vi "Read Detector Status.vi"(8 "Error In":errorcluster, 11 "KIT-QVA in":refnum<class "KIT-QVA.lvclass">) -> (0 "Error Out":errorcluster, 3 "KIT-QVA out":refnum<class "KIT-QVA.lvclass">)   [LabVIEW 2014, in "KIT-QVA.lvlib" / "KIT-QVA.lvclass"]
doc: "Read detector status and publish."
uses:
  KIT-QVA.lvclass
  KIT-QVA.lvclass/KIT-QVA.ctl
  instr.lib/KIT-QV/KIT QV.lvlib
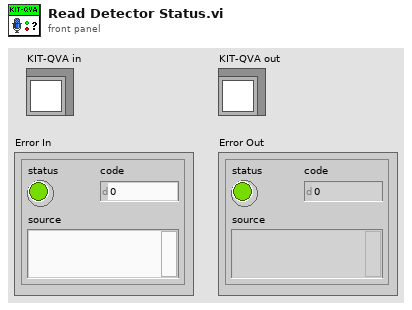
[diagram p1: front panel]
types:
  T1 = cluster{"System Test":bool, "Test Mode":bool, "Fault":bool, "Quench":bool, "U/T Fault":bool, "Bus Error":bool, "System Fault":bool, "Reserved":bool}
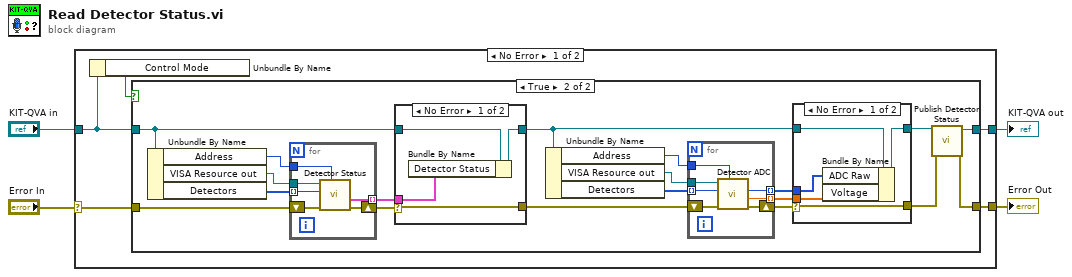
[diagram p0: block diagram]
diagram:
  n1 = case shown="No Error" "Error In" {
    selector: "Error In" -> [w7 w58]
    tunnel: [w8 w58] -> w3
    tunnel: [w9 w57] -> w1
    tunnel: "KIT-QVA in" -> [w6 w57]
    frame No Error {
      n2 = Unbundle By Name(w6) -> ("Control Mode"=w5:bool)
      n3 = case shown="True" w5 {
        tunnel: [w11 w30] -> w9
        tunnel: [w10 w29] -> w8
        tunnel: w7 -> [w10 w28]
        tunnel: w6 -> [w11 w12]
        frame False {
        }
        frame True {
          n4 = Unbundle By Name(w12) -> ("Address"=w25:u16, "VISA Resource out"=w26:refnum<visa-resource-name>, "Detectors"=w23:u8[])
          n5 = for {
            tunnel: w26 -> [w48]
            tunnel: w25 -> [w47]
            tunnel: [w46] -> w24 mode=indexing
            shift-right: [w49] -> w27
            shift-left: w28 -> [w50]
            tunnel: w23 -> [w45] mode=indexing
            n6 = call "Detector Status.vi"("Address"=w47, "Error In"=w50, "Detector"=w45, "VISA Resource in"=w48) -> ("Error Out"=w49:errorcluster, "Detector Cluster"=w46:T1)  [unwired: 4 in, 2 out]
          }
          n7 = case shown="No Error" w27 {
            selector: w27 -> [w51 w55]
            tunnel: w24 -> [w54 _]
            tunnel: w12 -> [w53 w56]
            tunnel: [w52 w56] -> w16
            tunnel: [w51 w55] -> w17
            frame No Error {
              n8 = Bundle By Name(cluster=w53, "Detector Status"=w54) -> (w52:refnum<class "KIT-QVA.lvclass">)
            }
            frame Error {
            }
          }
          n9 = Unbundle By Name(w16) -> ("Address"=w20:u16, "VISA Resource out"=w19:refnum<visa-resource-name>, "Detectors"=w22:u8[])
          n10 = for {
            tunnel: w19 -> [w36]
            tunnel: w20 -> [w37]
            tunnel: [w32] -> w21 mode=indexing
            shift-right: [w33] -> w18
            shift-left: w17 -> [w34]
            tunnel: w22 -> [w35] mode=indexing
            tunnel: [w31] -> w13 mode=indexing
            n11 = call "Detector ADC.vi"("Address"=w37, "Error In"=w34, "Detector"=w35, "VISA Resource in"=w36) -> ("Error Out"=w33:errorcluster, "Voltage"=w32:dbl[unit], "ADC Raw"=w31:i16)  [unwired: 4 in, 1 out]
          }
          n12 = case shown="No Error" w18 {
            selector: w18 -> [w39 w43]
            tunnel: w21 -> [w42 _]
            tunnel: w16 -> [w41 w44]
            tunnel: [w40 w44] -> w15
            tunnel: [w39 w43] -> w14
            tunnel: w13 -> [w38 _]
            frame No Error {
              n13 = Bundle By Name(cluster=w41, "ADC Raw"=w38, "Voltage"=w42) -> (w40:refnum<class "KIT-QVA.lvclass">)
            }
            frame Error {
            }
          }
          n14 = call "Publish Detector Status.vi"("Error In"=w14, "KIT-QVA in"=w15) -> ("Error Out"=w29:errorcluster, "KIT-QVA out"=w30:refnum<class "KIT-QVA.lvclass">)  [unwired: 8 in]
        }
      }
    }
    frame Error {
    }
  }
  "Error Out" <- w3
  "KIT-QVA out" <- w1
